vi "InitDevices.vi"(8 "error in":errorcluster, 11 "Session In":T2) -> (0 "error out":errorcluster, 2 "Raw Image":T1, 3 "Session Out":T2)   [LabVIEW 2014]
uses:
  <vilib>/userdefined/High Color/IMAQdx.ctl
  <vilib>/vision/Image Controls.llb/IMAQ Image.ctl
  <vilib>/vision/driver/NI_Vision_Acquisition_Software.lvlib
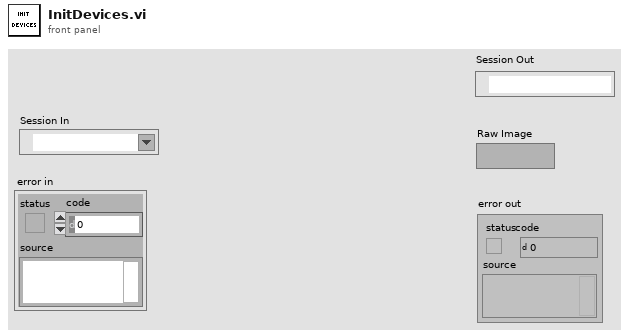
[diagram p1: front panel]
types:
  T1 = typedef "IMAQ Image.ctl" = refnum<image>
  T2 = typedef "IMAQdx.ctl" = refnum<k21>
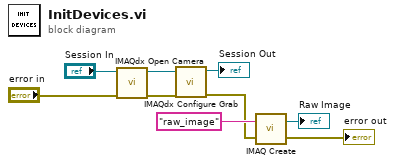
[diagram p0: block diagram]
diagram:
  n1 = call <vilib>:"IMAQdx Open Camera.vi"("error in"="error in", "Session In"="Session In") -> ("error out"=w7:errorcluster, "Session Out"=w6:T2)  [unwired: 8 in]
  n2 = call <vilib>:"IMAQdx Configure Grab.vi"("error in"=w7, "Session In"=w6) -> ("error out"=w3:errorcluster, "Session Out"=→"Session Out":T2)  [unwired: 8 in]
  n3 = call "IMAQ Create"("Image Name"="raw_image", "error in (no error)"=w3) -> ("New Image"=→"Raw Image":T1, "error out"=→"error out":errorcluster)  [unwired: 3 in]
